vi "load login credentials.vi"(8 "error in":errorcluster, 10 "Device Model":enum16{"cRIO-9068"}(ring)) -> (0 "error out":errorcluster, 1 "Password":string, 2 "Username":string, 3 "IP Address":string)   [LabVIEW 2016, in "SMI Tests.lvlib"]
uses:
  SMI Tests.lvlib
  <vilib>/Utility/config.llb/Read Key (String).vi
  <vilib>/Utility/config.llb/NI_LVConfig.lvlib
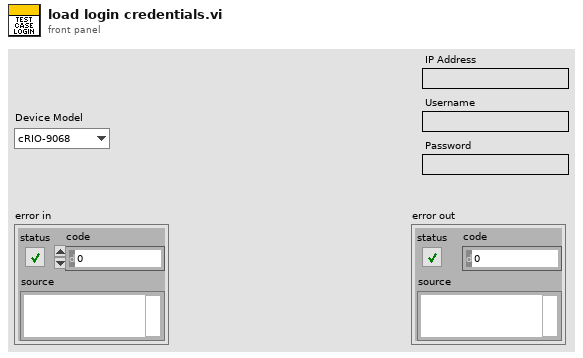
[diagram p1: front panel]
types:
  T1 = typedef "NI_LVConfig.lvlib/Config Data RefNum.ctl" = refnum<k1>
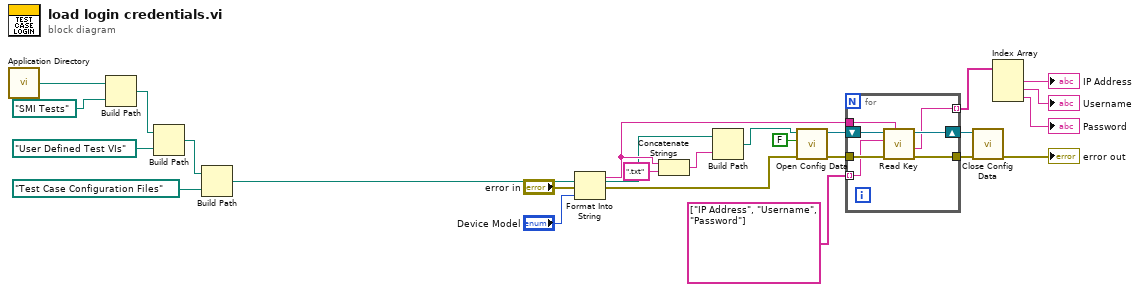
[diagram p0: block diagram]
diagram:
  n1 = call <vilib>:"Application Directory.vi"() -> ("Application Directory"=w7:path)
  n2 = Build Path(base path=w7, name or relative path=path "SMI Tests") -> (appended path=w5:path)
  n3 = Build Path(base path=w5, name or relative path=path "User Defined Test VIs") -> (appended path=w2:path)
  n4 = Build Path(base path=w2, name or relative path=path "Test Case Configuration Files") -> (appended path=w1:path)
  n5 = Format Into String(error in="error in", "Device Model") -> (resulting string=w9:string, error out=w23:errorcluster)  [unwired: 2 in]
  n6 = Concatenate Strings(w9, ".txt" ("string")) -> (w8:string)
  n7 = Build Path(base path=w1, name or relative path=w8) -> (appended path=w22:path)
  n8 = call <vilib>:"Open Config Data.vi"("error in (no error)"=w23, "create file if necessary (T)"=FALSE, "configuration file path"=w22) -> ("error out"=w19:errorcluster, "refnum"=w20:T1)  [unwired: 6 in, 1 out]
  n9 = for {
    tunnel: w19 -> [w31]
    tunnel: w9 -> [w30]
    tunnel: string[] ["IP Address", "Username", "Password"] -> [w29] mode=indexing
    shift-right: [w28] -> w15
    shift-left: w20 -> [w32]
    tunnel: [w27] -> w16
    tunnel: [w26] -> w14 mode=indexing
    n10 = call-poly <vilib>:"Read Key.vi"("section"=w30, "error in (no error)"=w31, "key"=w29, "refnum"=w32) -> ("error out"=w27:errorcluster, "value"=w26:string, "refnum out"=w28:T1)  [unwired: 4 in, 1 out]
  }
  n11 = call <vilib>:"Close Config Data.vi"("error in (no error)"=w16, "refnum"=w15) -> ("error out"=→"error out":errorcluster)  [unwired: 8 in, 1 out]
  n12 = Index Array(array=w14) -> (element #1=→"IP Address":string, element #2=→"Username":string, element #3=→"Password":string)  [unwired: 3 in]
